vi "GDSProject_GetProjectItem.vi"(0 "ProjectItemToSearchFrom":refnum<vi>, 5 "error in (no error)":errorcluster) -> (14 "ProjectItemToSearchFromOut":refnum<vi>, 15 "ItemFound":bool, 16 "ProjectItemFound":refnum<vi>, 19 "error out":errorcluster)   [LabVIEW 2020]
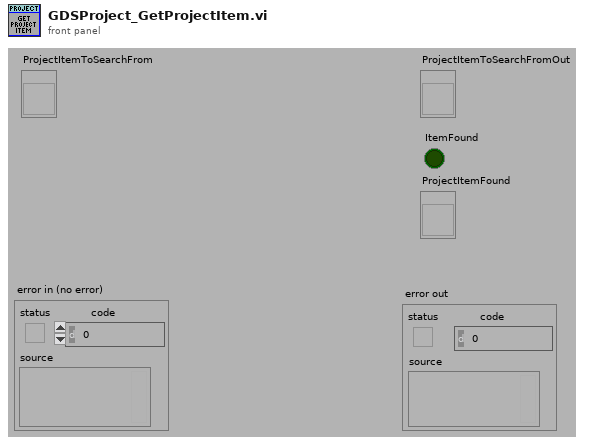
[diagram p1: front panel]
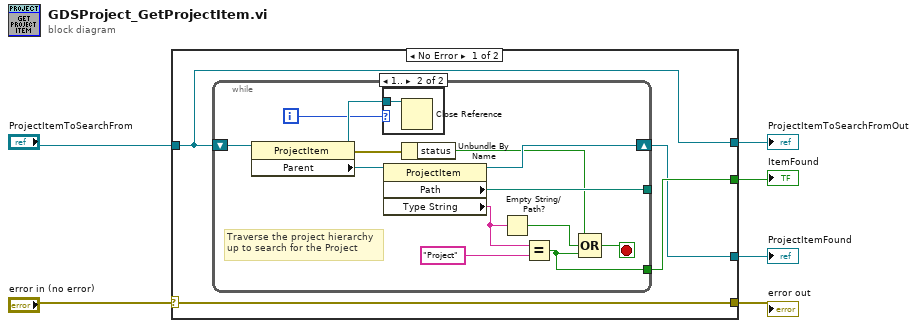
[diagram p0: block diagram]
diagram:
  n1 = case shown="No Error" "error in (no error)" {
    selector: "error in (no error)" -> [w7 w26]
    tunnel: [w7 w26] -> w5
    tunnel: "ProjectItemToSearchFrom" -> [w9 w25]
    tunnel: [w10 _] -> w3
    tunnel: [w9 w25] -> w2
    tunnel: [w8 _] -> w1
    frame No Error {
      n2 = while {
        shift-right: [w21] -> w8
        shift-left: w9 -> [w22]
        tunnel: [w18] -> _
        tunnel: [w11] -> w10
        i -> [w14]
        stop <- w20 stop-if-true
        # "Traverse the project hierarchy\nup to search for the Project"
        n3 = property class="ProjectItem"(reference=w22) -> (reference out=w15:refnum<vi>, error out=w17:errorcluster, "Parent"=w23:refnum<vi>)  [unwired: 1 in]
        n4 = case shown="1.." w14 {
          tunnel: w15 -> [_ w24]
          frame 0, Default {
          }
          frame 1.. {
            n5 = Close Reference(reference=w24) -> ()  [unwired: 1 in, 1 out]
          }
        }
        n6 = property class="ProjectItem"(reference=w23) -> (reference out=w21:refnum<vi>, "Path"=w18:path, "Type String"=w13:string)  [unwired: 1 in, 1 out]
        n7 = Unbundle By Name(w17) -> ("status"=w16:bool)
        n8 = Empty String/Path?(string/path=w13) -> (empty?=w12:bool)
        n9 = Equal?(x=w13, y="Project") -> (x = y?=w11:bool)
        n10 = Compound Arithmetic op=OR(w16, w12, w11) -> (w20:bool)
      }
    }
    frame Error {
    }
  }
  "error out" <- w5
  "ProjectItemToSearchFromOut" <- w2
  "ProjectItemFound" <- w1
  "ItemFound" <- w3
